vi "CreateLVAddonJSONfile.vi"   [LabVIEW 2021]
uses:
  <vilib>/Utility/sysdir.llb/System Directory Type.ctl
  <vilib>/Wiresmith Technology/G CLI/CLI Class/CLI.lvclass
types:
  T1 = typedef "System Directory Type.ctl" = i32
  T2 = enum32{"Invalid", "Standard", "Closed", "Hidden", "Minimized", "Maximized"}
  T3 = enum16{"open", "replace", "create", "open or create", "replace or create", "replace or create with confirmation"}
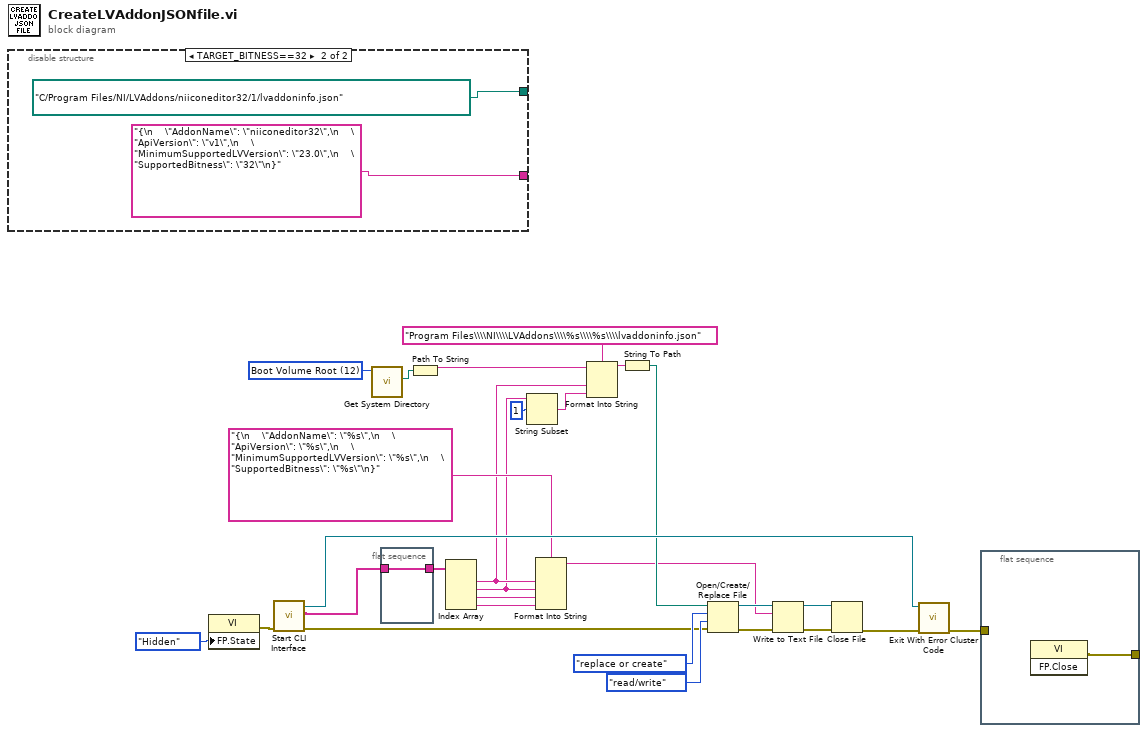
[diagram p0: block diagram]
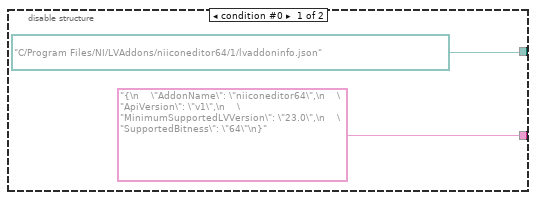
[diagram p2: hidden frame]
diagram:
  w11 = T1 12 items=["User Home"=0, "User Desktop"=1, "User Documents"=2, "User Application Data"=3, "User Preferences"=4, "User Temporary"=5, "Public Documents"=6, "Public Application Data"=7, "Public Preferences"=8, "Public Cache"=13, "System Core Libraries"=9, "System Installed Libraries"=10, "Application Files"=11, "Boot Volume Root"=12] ("system directory type")
  n1 = disable-structure shown="TARGET_BITNESS==32" {
    disable-tunnel: [path "C:/Program Files/NI/LVAddons/niiconeditor64/1/lvaddoninfo.json" ("Destination[i] Paths (Absolute)") path "C:/Program Files/NI/LVAddons/niiconeditor32/1/lvaddoninfo.json" ("Destination[i] Paths (Absolute)")] -> _
    disable-tunnel: ["{\n    \"AddonName\": \"niiconeditor64\",\n    \"ApiVersion\": \"v1\",\n    \"MinimumSupportedLVVersion\": \"23.0\",\n    \"SupportedBitness\": \"64\"\n}" ("Tag Name") "{\n    \"AddonName\": \"niiconeditor32\",\n    \"ApiVersion\": \"v1\",\n    \"MinimumSupportedLVVersion\": \"23.0\",\n    \"SupportedBitness\": \"32\"\n}" ("Tag Name")] -> _
    frame condition #0 {
    }
    frame condition #1 (active) {
    }
  }
  n2 = property class="VI"("FP.State"=T2."Hidden" ("Front Panel Window:State")) -> (error out=w21:errorcluster)  [unwired: 2 in, 1 out]
  n3 = call <vilib>:"Start CLI Interface.vi"("error in (no error)"=w21) -> ("error out"=w17:errorcluster, "Custom Parameters"=w16:string[], "CLI out"=w19:refnum<class "CLI.lvclass">)  [unwired: 7 in, 1 out]
  n4 = call <vilib>:"Get System Directory.vi"("system directory type"=w11) -> ("system directory"=w3:path)  [unwired: 10 in]
  n5 = flat-sequence {
    tunnel: w16 -> [w33]
    tunnel: [w33] -> w15
    frame #0 {
    }
  }
  n6 = Path To String(path=w3) -> (string=w2:string)
  n7 = Index Array(array=w15) -> (element #1=w9:string, element #2=w8:string, element #3=w14:string, element #4=w13:string)  [unwired: 4 in]
  n8 = String Subset(string=w8, offset (0)=1) -> (substring=w6:string)  [unwired: 1 in]
  n9 = Format Into String(format string="{\n    \"AddonName\": \"%s\",\n    \"ApiVersion\": \"%s\",\n    \"MinimumSupportedLVVersion\": \"%s\",\n    \"SupportedBitness\": \"%s\"\n}" ("Tag Name"), w9, w8, w14, w13) -> (resulting string=w1:string)  [unwired: 2 in, 1 out]
  n10 = Format Into String(format string="Program Files\\\\NI\\\\LVAddons\\\\%s\\\\%s\\\\lvaddoninfo.json", initial string=w2, w9, w6) -> (resulting string=w5:string)  [unwired: 1 in, 1 out]
  n11 = String To Path(string=w5) -> (path=w4:path)
  n12 = Open/Create/Replace File(file path (use dialog)=w4, error in=w17, operation (0:open)=T3."replace or create", access (0:read/write)=enum16{"read/write", "read-only", "write-only"}."read/write") -> (refnum out=w27:refnum<file>, error out=w24:errorcluster)  [unwired: 2 in, 1 out]
  n13 = Write to Text File(file (use dialog)=w27, text=w1, error in=w24) -> (refnum out=w28:refnum<file>, error out=w23:errorcluster)  [unwired: 1 in, 1 out]
  n14 = Close File(refnum=w28, error in=w23) -> (error out=w20:errorcluster)  [unwired: 1 out]
  n15 = call <vilib>:"Exit With Error Cluster Code.vi"("error in (no error)"=w20, "CLI in"=w19) -> ("error out"=w18:errorcluster)  [unwired: 9 in]
  n16 = flat-sequence {
    tunnel: [w34] -> _
    tunnel: w18 -> [_]
    frame #0 {
      n17 = invoke class="VI" method="FP.Close"() -> (error out=w34:errorcluster)  [unwired: 3 in, 2 out]
    }
  }
